vi "SingleLineRead.vi"(6 "Sim":bool, 7 "line":string, 8 "Holder Length":dbl format="%#_13g") -> (0 "InRange":bool, 1 "length":dbl, 2 "armAngle":i32, 3 "baseAngle":i32, 5 "error out":errorcluster)   [LabVIEW 2013]
panel:
  out "XY Graph":cluster{"X":dbl, "Y":dbl}[](graph)
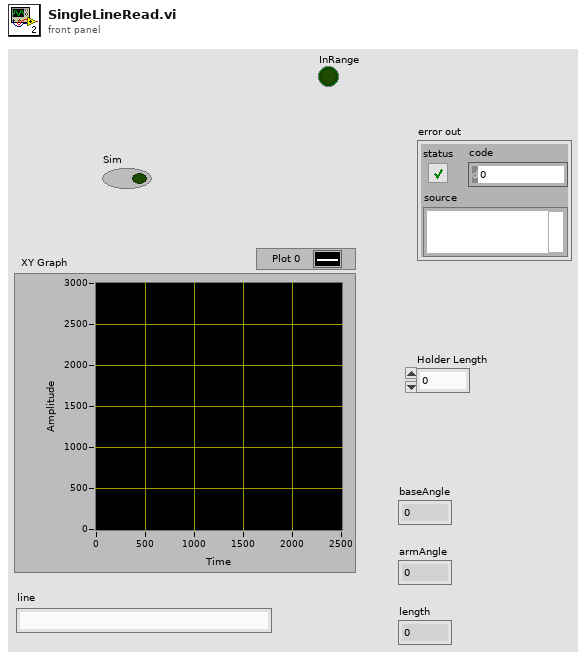
[diagram p1: front panel]
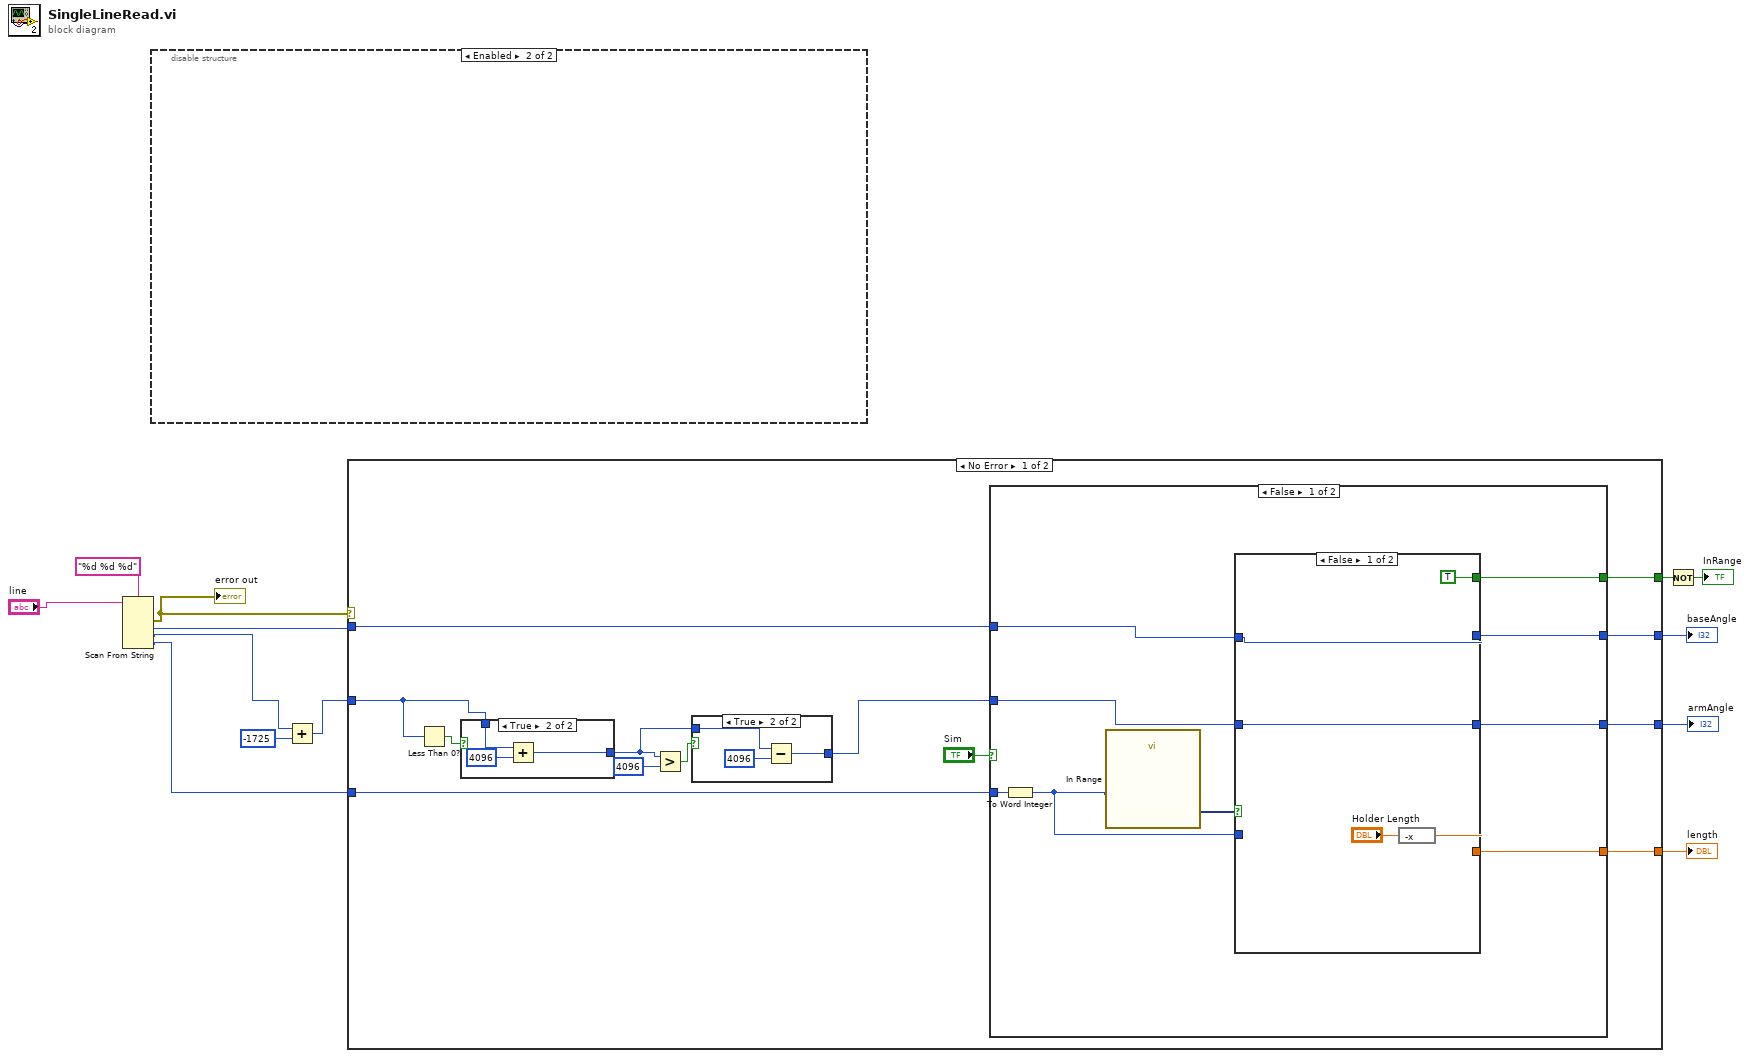
[diagram p0: block diagram]
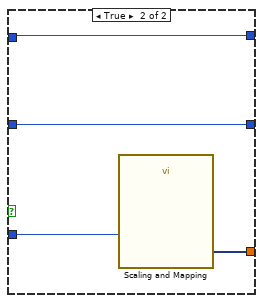
[diagram p4: hidden frame]
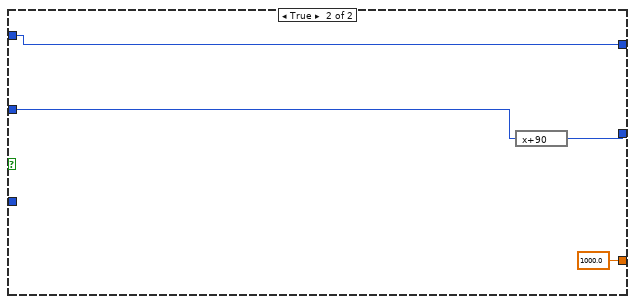
[diagram p5: hidden frame]
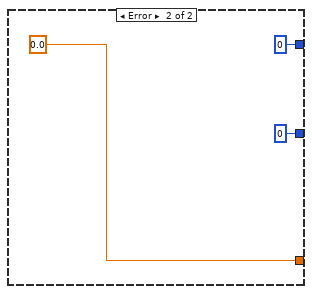
[diagram p6: hidden frame]
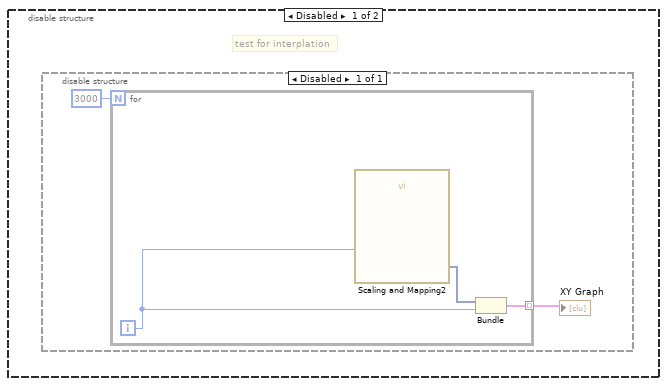
[diagram p7: hidden frame]
diagram:
  n1 = Scan From String(format string="%d %d %d", input string="line") -> (error out=w7:errorcluster, output 1=w8:i32, output 2=w2:i32, output 3=w9:i32)  [unwired: 5 in, 2 out]
  "error out" <- w7
  n2 = disable-structure shown="Enabled" {
    frame Disabled {
      # "test for interplation"
      n3 = disable-structure shown="Disabled" {
        frame Disabled {
          n4 = for {
            N: 3000 -> [_]
            tunnel: [w16] -> w14 mode=indexing
            i -> [w17]
            n5 = call "Scaling and Mapping2"("Signals"=w17) -> ("Scaled Signals"=w18:dynamicdata)  [unwired: 9 in, 1 out]
            n6 = Bundle("Scaled Signals"=w18, w17) -> (w16:cluster{"Scaled Signals":dynamicdata, i32})  [unwired: 1 in]
          }
          "XY Graph" <- w14
        }
      }
    }
    frame Enabled {
    }
  }
  n7 = Add(x=w2, y=-1725) -> (x+y=w1:i32)
  n8 = case shown="No Error" w7 {
    tunnel: [w31 0.0] -> w13
    tunnel: w8 -> [w30 _]
    tunnel: w1 -> [w20 _]
    tunnel: w9 -> [w28 _]
    tunnel: [w27 _] -> w12
    tunnel: [w26 0] -> w5
    tunnel: [w25 0] -> w4
    frame No Error {
      n9 = Less Than 0?(x=w20) -> (x < 0?=w24:bool)
      n10 = case shown="True" w24 {
        tunnel: w20 -> [w36 w39]
        tunnel: [w36 w37] -> w21
        frame False {
        }
        frame True {
          n11 = Add(x=w39, y=4096) -> (x+y=w37:i32)
        }
      }
      n12 = Greater?(x=w21, y=4096) -> (0:w22:bool)
      n13 = case shown="True" w22 {
        tunnel: w21 -> [w32 w35]
        tunnel: [w32 w33] -> w19
        frame False {
        }
        frame True {
          n14 = Subtract(x=w35, y=4096) -> (x-y=w33:i32)
        }
      }
      n15 = case shown="False" "Sim" {
        tunnel: [w48 1000.0] -> w31
        tunnel: w28 -> [w43 _]
        tunnel: [w47 w61] -> w26
        tunnel: w30 -> [w46 w61]
        tunnel: w19 -> [w45 w59]
        tunnel: [w44 w60] -> w25
        tunnel: [w42 _] -> w27
        frame False {
          n16 = To Word Integer(number=w43) -> (16bit integer=w41:i16)
          n17 = call "In Range"("Operand 1"=w41) -> ("Result"=w40:dynamicdata)  [unwired: 9 in, 1 out]
          n18 = case shown="False" w40 {
            tunnel: [w49 w57] -> w48
            tunnel: w41 -> [_ w56]
            tunnel: w46 -> [w52 w55]
            tunnel: [w52 w55] -> w47
            tunnel: w45 -> [w51 w54]
            tunnel: [w51 w54] -> w44
            tunnel: [TRUE _] -> w42
            frame False {
              n19 = expression code="-x"("Holder Length") -> (w49:dbl)
            }
            frame True {
              n20 = call "Scaling and Mapping"("Signals"=w56) -> ("Scaled Signals"=w57:dynamicdata)  [unwired: 9 in, 1 out]
            }
          }
        }
        frame True {
          n21 = expression code="x+90"(w59) -> (w60:i32)
        }
      }
    }
    frame Error {
    }
  }
  "baseAngle" <- w5
  "armAngle" <- w4
  "length" <- w13
  n22 = Not(x=w12) -> (.not. x?=→"InRange":bool)
